vi "Write Polling Interval Minimum.vi"(8 "error in (no error)":errorcluster, 10 "Polling Interval Minimum":dbl[unit]=-1.0, 11 "CS++BaseActor in":refnum<class "CS++BaseActor.lvclass">) -> (0 "error out":errorcluster, 3 "CS++BaseActor out":refnum<class "CS++BaseActor.lvclass">)   [LabVIEW 2015, in "CS++BaseActor.lvlib" / "CS++BaseActor.lvclass"]
doc: "Write minum time interval for polling using Time-Delayed Message."
uses:
  CS++BaseActor.lvclass
  CS++BaseActor.lvclass/CS++BaseActor.ctl
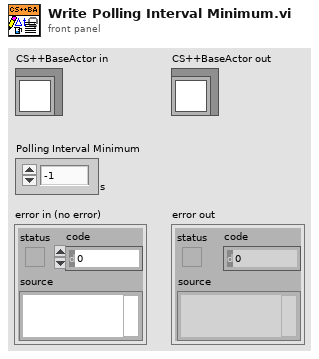
[diagram p1: front panel]
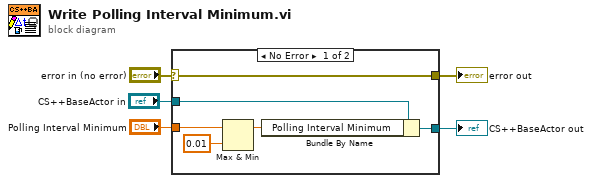
[diagram p0: block diagram]
diagram:
  n1 = case shown="No Error" "error in (no error)" {
    selector: "error in (no error)" -> [w11 w12]
    tunnel: [w11 w12] -> w4
    tunnel: [w9 w13] -> w2
    tunnel: "CS++BaseActor in" -> [w10 w13]
    tunnel: "Polling Interval Minimum" -> [w8 _]
    frame No Error {
      n2 = Max & Min(x=w8, y=dbl[unit] 0.01) -> (max(x,y)=w7:dbl[unit])  [unwired: 1 out]
      n3 = Bundle By Name(cluster=w10, "Polling Interval Minimum"=w7) -> (w9:refnum<class "CS++BaseActor.lvclass">)
    }
    frame Error {
    }
  }
  "error out" <- w4
  "CS++BaseActor out" <- w2
